vi "WPI_SolenoidClose.vi"(8 "error in (no error)":errorcluster, 11 "SolenoidDevRef":T1={"DevStatus"={"status"=FALSE, "code"=0, "source"=""}, "Pneumatics Control Module"=0, "Forward Solenoid Channel"=enum."Invalid", "Reverse Solenoid Channel"=enum."Invalid"}) -> (0 "error out":errorcluster)   [LabVIEW 2017]
doc: "Closes the reference to the solenoid you specify. Use this VI to close each solenoid reference that you open with the Open VI.\n\nThis software is licensed. Open the labview\\readme\\WPI Robotics Library Open Source License.txt file for more information."
uses:
  <vilib>/Rock Robotics/WPI/Solenoid/WPI_SolenoidDevRef.ctl
  <vilib>/Rock Robotics/WPI/Solenoid/WPI_SolenoidChannel.ctl
  <vilib>/Rock Robotics/WPI/Solenoid/WPI_SolenoidCacheOp.ctl
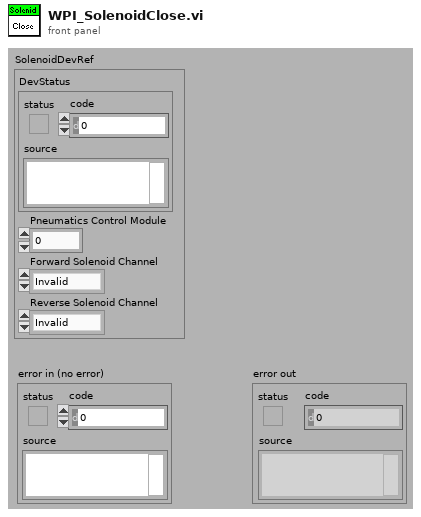
[diagram p1: front panel]
types:
  T1 = typedef "WPI_SolenoidDevRef.ctl" = cluster{"DevStatus":errorcluster, "Pneumatics Control Module":u8, "Forward Solenoid Channel":T2, "Reverse Solenoid Channel":T2}
  T2 = typedef "WPI_SolenoidChannel.ctl" = enum8{"Solenoid 0", "Solenoid 1", "Solenoid 2", "Solenoid 3", "Solenoid 4", "Solenoid 5", "Solenoid 6", "Solenoid 7", "Invalid"}
  T3 = typedef "WPI_SolenoidCacheOp.ctl" = enum16{"Acquire", "Release", "Status"}
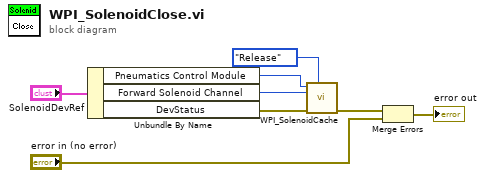
[diagram p0: block diagram]
diagram:
  n1 = Unbundle By Name("SolenoidDevRef") -> ("Pneumatics Control Module"=w5:u8, "Forward Solenoid Channel"=w7:T2, "DevStatus"=w6:errorcluster)
  n2 = call <vilib>:"WPI_SolenoidCache.vi"("AllocatedSolenoidOp"=WPI_SolenoidCacheOp."Release", "error in (no error)"=w6, "SolenoidChannel"=w7, "Pneumatics Control Module"=w5) -> ("error out"=w3:errorcluster)  [unwired: 1 in, 6 out]
  n3 = Merge Errors(w3, "error in (no error)") -> (→"error out":errorcluster)
